vi "FTW-JSON-Object-SetElement-Object.vi"(0 "JSON Object":refnum<class "FTW-JSON.lvclass">, 5 "Key":string, 11 "error in":errorcluster) -> (4 "JSON Root Object":refnum<class "FTW-JSON.lvclass">, 6 "JSON Sub-Object":refnum<class "FTW-JSON.lvclass">, 15 "error out":errorcluster)   [LabVIEW 2013, in "FTW-JSON.lvclass"]
uses:
  FTW-JSON.lvclass
  FTW-JSON.lvclass/FTW-JSON.ctl
panel:
  # "Inputs"
  # "Outputs"
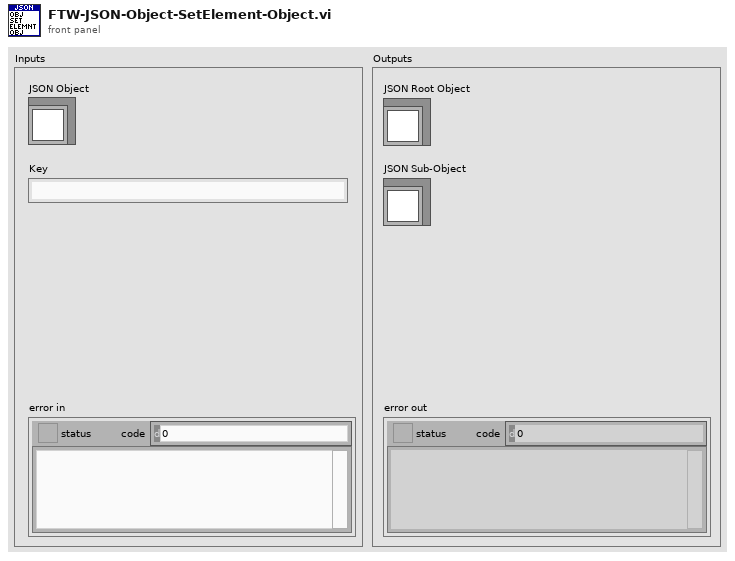
[diagram p1: front panel]
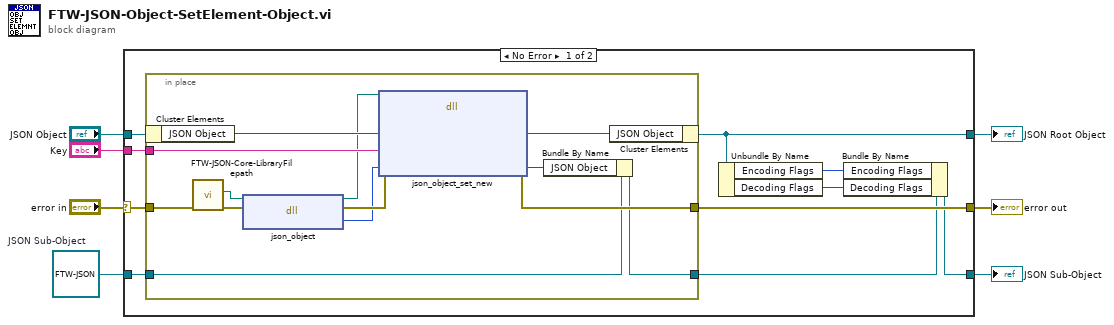
[diagram p0: block diagram]
diagram:
  w1 = refnum<class "FTW-JSON.lvclass"> refnum  # JSON Sub-Object
  n1 = case shown="No Error" "error in" {
    selector: "error in" -> [w17 w33]
    tunnel: [w16 w33] -> w7
    tunnel: [w11 w32] -> w5
    tunnel: "JSON Object" -> [w15 w32]
    tunnel: "Key" -> [w14 _]
    tunnel: [w10 w31] -> w2
    tunnel: w1 -> [w12 w31]
    frame No Error {
      n2 = in-place {
        in-place-border: w17 -> [w30]
        in-place-border: [w29] -> w16
        in-place-border: w14 -> [w26]
        in-place-border: [w19] -> w13
        in-place-border: w12 -> [w20]
        n3 = in-place-cluster #1(w15) -> ("JSON Object"=w28:i64)
        n4 = call "FTW-JSON-Core-LibraryFilepath.vi"("error in"=w30) -> ("error out"=w23:errorcluster, "JSON Library Filepath"=w25:path)  [unwired: 9 in]
        n5 = dll-call lib="?" fn="json_object"(path in=w25, error in=w23) -> (path out=w24:path, error out=w22:errorcluster, "New Object"=w21:i64)  [unwired: 1 in]
        n6 = dll-call lib="?" fn="json_object_set_new"(path in=w24, error in=w22, "JSON Object Pointer"=w28, "Key"=w26, "New JSON Object"=w21) -> (error out=w29:errorcluster, "JSON Object Pointer"=w27:i64, "New JSON Object"=w18:i64)  [unwired: 3 in, 1 out]
        n7 = Bundle By Name(cluster=w20, "JSON Object"=w18) -> (w19:refnum<class "FTW-JSON.lvclass">)
        n8 = in-place-cluster #1("JSON Object"=w27) -> (w11:refnum<class "FTW-JSON.lvclass">)
      }
      n9 = Unbundle By Name(w11) -> ("Encoding Flags"=w9:i64, "Decoding Flags"=w8:i64)
      n10 = Bundle By Name(cluster=w13, "Encoding Flags"=w9, "Decoding Flags"=w8) -> (w10:refnum<class "FTW-JSON.lvclass">)
    }
    frame Error {
    }
  }
  "error out" <- w7
  "JSON Root Object" <- w5
  "JSON Sub-Object" <- w2
